vi "Swerve Drive.vi"(6 "Field Centric?":bool, 7 "Cluster":T1, 9 "Robot Velocities":T12, 10 "PigeonIMUDevRef":T10 {"Type" items=["CAN"=352321536, "TalonSRX"=33554432]}, 11 "Motors":T2={"Drive Motors"={"Motor Type"=enum."Falcon 500", "Motors"={"Left Front"={"DeviceStatus"={"status"=FALSE, "code"=0, "source"=""}, "Type"=enum."PWM", "PWM"={"PWM Channel"=enum."PWM 0", "DeadBand"={"Name"="", "maxPositivePwm"=0, "minPositivePwm"=0, "centerPwm"=0, "maxNegativePwm"=0, "minNegativePwm"=0, "angularRange"=0}}, "CAN"={"Device Number"=0, "SetOutput VI Ref"=variant, "GetOutput VI Ref"=variant, "Enable VI Ref"=variant, "Disable VI Ref"=variant, "Data"=variant}, "Invert"=FALSE, "DIO PWM"={"PWM \"Enable\" Channel"=enum."PWM 0", "DIOChannel"=enum."DIO 0", "PWM Rate"=0.0}}, "Left Back"={"DeviceStatus"={"status"=FALSE, "code"=0, "source"=""}, "Type"=enum."PWM", "PWM"={"PWM Channel"=enum."PWM 0", "DeadBand"={"Name"="", "maxPositivePwm"=0, "minPositivePwm"=0, "centerPwm"=0, "maxNegativePwm"=0, "minNegativePwm"=0, "angularRange"=0}}, "CAN"={"Device Number"=0, "SetOutput VI Ref"=variant, "GetOutput VI Ref"=variant, "Enable VI Ref"=variant, "Disable VI Ref"=variant, "Data"=variant}, "Invert"=FALSE, "DIO PWM"={"PWM \"Enable\" Channel"=enum."PWM 0", "DIOChannel"=enum."DIO 0", "PWM Rate"=0.0}}, "Right Front"={"DeviceStatus"={"status"=FALSE, "code"=0, "source"=""}, "Type"=enum."PWM", "PWM"={"PWM Channel"=enum."PWM 0", "DeadBand"={"Name"="", "maxPositivePwm"=0, "minPositivePwm"=0, "centerPwm"=0, "maxNegativePwm"=0, "minNegativePwm"=0, "angularRange"=0}}, "CAN"={"Device Number"=0, "SetOutput VI Ref"=variant, "GetOutput VI Ref"=variant, "Enable VI Ref"=variant, "Disable VI Ref"=variant, "Data"=variant}, "Invert"=FALSE, "DIO PWM"={"PWM \"Enable\" Channel"=enum."PWM 0", "DIOChannel"=enum."DIO 0", "PWM Rate"=0.0}}, "Right Back"={"DeviceStatus"={"status"=FALSE, "code"=0, "source"=""}, "Type"=enum."PWM", "PWM"={"PWM Channel"=enum."Invalid", "DeadBand"={"Name"="", "maxPositivePwm"=0, "minPositivePwm"=0, "centerPwm"=0, "maxNegativePwm"=0, "minNegativePwm"=0, "angularRange"=0}}, "CAN"={"Device Number"=0, "SetOutput VI Ref"=variant, "GetOutput VI Ref"=variant, "Enable VI Ref"=variant, "Disable VI Ref"=variant, "Data"=variant}, "Invert"=FALSE, "DIO PWM"={"PWM \"Enable\" Channel"=enum."Invalid", "DIOChannel"=enum."Invalid", "PWM Rate"=0.0}}}}, "Steering Motors"={"Motor Type"=enum."Falcon 500", "Motors"={"Left Front"={"DeviceStatus"={"status"=FALSE, "code"=0, "source"=""}, "Type"=enum."PWM", "PWM"={"PWM Channel"=enum."PWM 0", "DeadBand"={"Name"="", "maxPositivePwm"=0, "minPositivePwm"=0, "centerPwm"=0, "maxNegativePwm"=0, "minNegativePwm"=0, "angularRange"=0}}, "CAN"={"Device Number"=0, "SetOutput VI Ref"=variant, "GetOutput VI Ref"=variant, "Enable VI Ref"=variant, "Disable VI Ref"=variant, "Data"=variant}, "Invert"=FALSE, "DIO PWM"={"PWM \"Enable\" Channel"=enum."PWM 0", "DIOChannel"=enum."DIO 0", "PWM Rate"=0.0}}, "Left Back"={"DeviceStatus"={"status"=FALSE, "code"=0, "source"=""}, "Type"=enum."PWM", "PWM"={"PWM Channel"=enum."PWM 0", "DeadBand"={"Name"="", "maxPositivePwm"=0, "minPositivePwm"=0, "centerPwm"=0, "maxNegativePwm"=0, "minNegativePwm"=0, "angularRange"=0}}, "CAN"={"Device Number"=0, "SetOutput VI Ref"=variant, "GetOutput VI Ref"=variant, "Enable VI Ref"=variant, "Disable VI Ref"=variant, "Data"=variant}, "Invert"=FALSE, "DIO PWM"={"PWM \"Enable\" Channel"=enum."PWM 0", "DIOChannel"=enum."DIO 0", "PWM Rate"=0.0}}, "Right Front"={"DeviceStatus"={"status"=FALSE, "code"=0, "source"=""}, "Type"=enum."PWM", "PWM"={"PWM Channel"=enum."PWM 0", "DeadBand"={"Name"="", "maxPositivePwm"=0, "minPositivePwm"=0, "centerPwm"=0, "maxNegativePwm"=0, "minNegativePwm"=0, "angularRange"=0}}, "CAN"={"Device Number"=0, "SetOutput VI Ref"=variant, "GetOutput VI Ref"=variant, "Enable VI Ref"=variant, "Disable VI Ref"=variant, "Data"=variant}, "Invert"=FALSE, "DIO PWM"={"PWM \"Enable\" Channel"=enum."PWM 0", "DIOChannel"=enum."DIO 0", "PWM Rate"=0.0}}, "Right Back"={"DeviceStatus"={"status"=FALSE, "code"=0, "source"=""}, "Type"=enum."PWM", "PWM"={"PWM Channel"=enum."Invalid", "DeadBand"={"Name"="", "maxPositivePwm"=0, "minPositivePwm"=0, "centerPwm"=0, "maxNegativePwm"=0, "minNegativePwm"=0, "angularRange"=0}}, "CAN"={"Device Number"=0, "SetOutput VI Ref"=variant, "GetOutput VI Ref"=variant, "Enable VI Ref"=variant, "Disable VI Ref"=variant, "Data"=variant}, "Invert"=FALSE, "DIO PWM"={"PWM \"Enable\" Channel"=enum."Invalid", "DIOChannel"=enum."Invalid", "PWM Rate"=0.0}}}}}) -> ()   [LabVIEW 2020]
uses:
  <vilib>/Rock Robotics/Network Tables/NT Write Numeric Array.vi
  Swerve Robot Project Template/Framework/Robot Global Data.vi
  Swerve Robot Project Template/Drive/Implementation/Robot Velocities.ctl
  <vilib>/Rock Robotics/WPI/ThirdParty/Phoenix-LabVIEW/Pigeon IMU/CTRE_PigeonIMU_ConnectionType.ctl
  <vilib>/Rock Robotics/WPI/ThirdParty/Phoenix-LabVIEW/Pigeon IMU/CTRE_PigeonIMU_DeviceRef.ctl
  <vilib>/Rock Robotics/SystemInterfaces/DIO/FPGA_DIOPWMChannel.ctl
  <vilib>/Rock Robotics/WPI/PWM/WPI_PWMDeadband.ctl
  <vilib>/Rock Robotics/WPI/MotorControl/WPI_MotorControlType.ctl
  <vilib>/Rock Robotics/SystemInterfaces/DIO/FPGA_DIOChannel.ctl
  <vilib>/Rock Robotics/WPI/MotorControl/WPI_MotorControlDeviceRef.ctl
  ctl/4 Motor Set.ctl
  ctl/Swerve Motors.ctl
  ctl/Motor Type.ctl
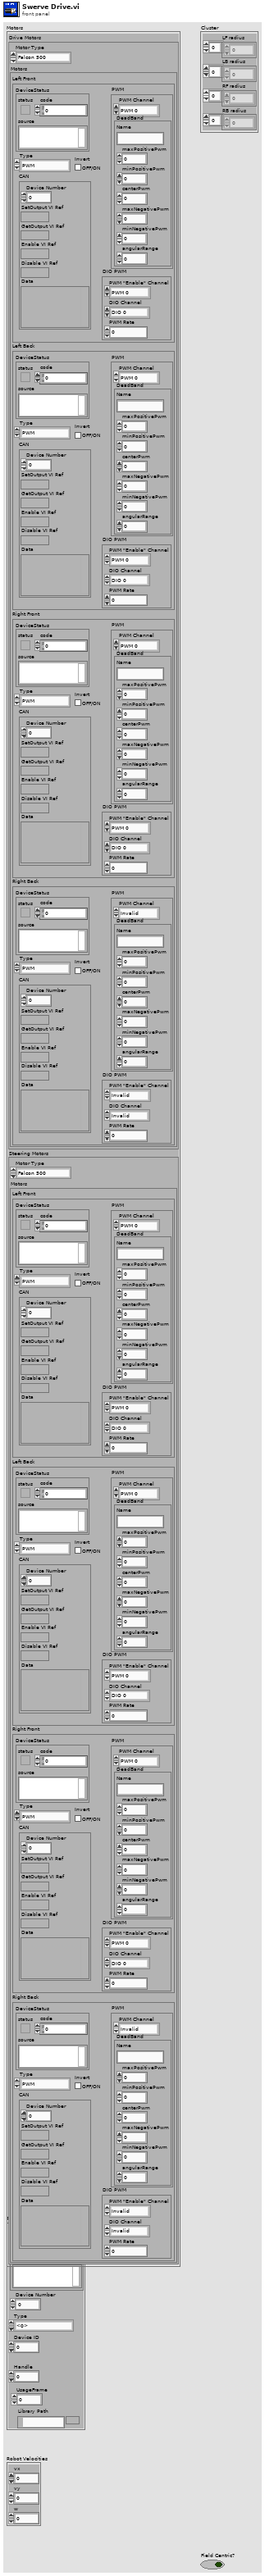
[diagram p1: front panel]
types:
  T1 = cluster{"LF radius":dbl[], "LB radius":dbl[], "RF radius":dbl[], "RB radius":dbl[]}
  T2 = typedef "Swerve Motors.ctl" = cluster{"Drive Motors":T3, "Steering Motors":T3}
  T3 = typedef "4 Motor Set.ctl" = cluster{"Motor Type":T4, "Motors":cluster{"Left Front":T5, "Left Back":T5, "Right Front":T5, "Right Back":T5}}
  T4 = typedef "Motor Type.ctl" = enum16{"Falcon 500", "NEO", "NEO 550"}
  T5 = typedef "WPI_MotorControlDeviceRef.ctl" = cluster{"DeviceStatus":errorcluster, "Type":T6, "PWM":cluster{"PWM Channel":T7, "DeadBand":T8}, "CAN":cluster{"Device Number":u8, "SetOutput VI Ref":variant, "GetOutput VI Ref":variant, "Enable VI Ref":variant, "Disable VI Ref":variant, "Data":variant}, "Invert":bool, "DIO PWM":cluster{"PWM \"Enable\" Channel":T7, "DIOChannel":T9, "PWM Rate":dbl}}
  T6 = typedef "WPI_MotorControlType.ctl" = enum16{"PWM", "CAN", "DIO PWM"}
  T7 = typedef "FPGA_DIOPWMChannel.ctl" = enum8{"PWM 0", "PWM 1", "PWM 2", "PWM 3", "PWM 4", "PWM 5", "PWM 6", "PWM 7", "PWM 8", "PWM 9", "PWM MXP 0", "PWM MXP 1", "PWM MXP 2", "PWM MXP 3", "PWM MXP 4", "PWM MXP 5", "PWM MXP 6", "PWM MXP 7", "PWM MXP 8", "PWM MXP 9", "Invalid"}
  T8 = typedef "WPI_PWMDeadband.ctl" = cluster{"Name":string, "maxPositivePwm":i32, "minPositivePwm":i32, "centerPwm":i32, "maxNegativePwm":i32, "minNegativePwm":i32, "angularRange":u16}
  T9 = typedef "FPGA_DIOChannel.ctl" = enum8{"DIO 0", "DIO 1", "DIO 2", "DIO 3", "DIO 4", "DIO 5", "DIO 6", "DIO 7", "DIO 8", "DIO 9", "DIO MXP 0", "DIO MXP 1", "DIO MXP 2", "DIO MXP 3", "DIO MXP 4", "DIO MXP 5", "DIO MXP 6", "DIO MXP 7", "DIO MXP 8", "DIO MXP 9", "DIO MXP 10", "DIO MXP 11", "DIO MXP 12", "DIO MXP 13", "DIO MXP 14", "DIO MXP 15", "SPI Port CS1", "SPI Port CS2", "SPI Port CS3", "SPI Port MISO", "SPI Port MOSI", "Invalid"}
  T10 = typedef "CTRE_PigeonIMU_DeviceRef.ctl" = cluster{"DeviceStatus":errorcluster, "Device Number":u8, "Type":T11, "Device ID":u32, "Handle":u64, "UsageFrame":u32, "Library Path":path}
  T11 = typedef "CTRE_PigeonIMU_ConnectionType.ctl" = u32
  T12 = typedef "Robot Velocities.ctl" = cluster{"vx":dbl, "vy":dbl, "w":dbl}
  T13 = cluster{"Left Front":dbl, "Left Back":dbl, "Right Front":dbl, "Right Back":dbl}
  T14 = typedef "Pod Setpoints.ctl" = cluster{"Left Front":cluster{"Velocity":dbl, "Theta":dbl}, "Left Back":cluster{"Velocity":dbl, "Theta":dbl}, "Right Front":cluster{"Velocity":dbl, "Theta":dbl}, "Right Back":cluster{"Velocity":dbl, "Theta":dbl}}
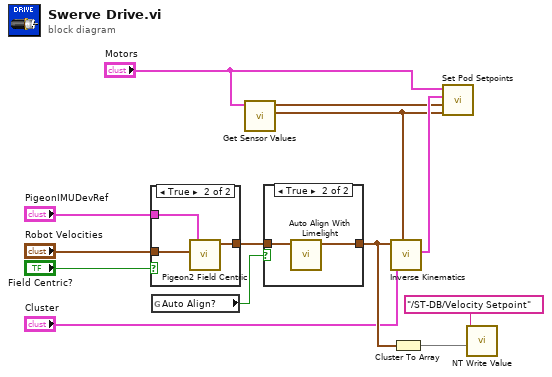
[diagram p0: block diagram]
diagram:
  n1 = case shown="True" "Field Centric?" {
    tunnel: "PigeonIMUDevRef" -> [_ w17]
    tunnel: "Robot Velocities" -> [w14 w16]
    tunnel: [w14 w15] -> w12
    frame False {
    }
    frame True {
      n2 = call "Pigeon2 Field Centric.vi"("Field Centric Velocities"=w16, "PigeonIMUDevRef"=w17) -> ("Robot Centric Velocities"=w15:T12)  [unwired: 9 in]
    }
  }
  n3 = global read "Robot Global Data.vi" "Auto Align?"() -> (w11:bool)
  n4 = call "Get Sensor Values.vi"("Motors"="Motors") -> ("Steer Angles (degrees)"=w4:T13, "Drive Velocities (ft/s)"=w3:T13)  [unwired: 7 in, 2 out]
  n5 = case shown="True" w11 {
    tunnel: w12 -> [w18 w20]
    tunnel: [w18 w19] -> w13
    frame False {
    }
    frame True {
      n6 = call "Auto Align With Limelight.vi"("Robot Velocities In"=w20) -> ("Robot Velocities Out"=w19:T12)  [unwired: 8 in, 1 out]
    }
  }
  n7 = call "Inverse Kinematics.vi"("Current Pod Steering (deg)"=w4, "Radii (ft)"="Cluster", "Target Velocity (ft/s and deg/s)"=w13) -> ("Pod Setpoints (ft/s and deg)"=w5:T14)  [unwired: 6 in, 2 out]
  n8 = Cluster To Array(cluster=w13) -> (array=w7:dbl[])
  n9 = call "Set Pod Setpoints.vi"("Steer Angles (degrees)"=w4, "Drive Velocities (ft/s)"=w3, "Pod Setpoints (ft/s and deg)"=w5, "Motors"="Motors") -> ()  [unwired: 8 in]
  n10 = call-poly <vilib>:"NT Write Value.vi"("value"=w7, "name"="/ST-DB/Velocity Setpoint" ("Name")) -> ()  [unwired: 9 in, 1 out]
